vi "SaveCoords.vi"(9 "Epoch Tel":dbl=2008.731741 caption="Époque" format="%.2f", 10 "DEC Tel":dbl=70342.56719999999 caption="Ascension Droite du Télescope" format="%<%H:%M:%S%1u>t", 11 "RA Tel":dbl=70342.56719999999 caption="Ascension Droite du Télescope" format="%<%H:%M:%S%1u>t") -> (0 "Accepted?":bool, 1 "Epoch Out":dbl=2008.731741 caption="Époque" format="%.2f", 2 "DEC Out":dbl=70342.56719999999 caption="Ascension Droite du Télescope" format="%<%H:%M:%S%1u>t", 3 "RA Out":dbl=70342.56719999999 caption="Ascension Droite du Télescope" format="%<%H:%M:%S%1u>t")   [LabVIEW 2019]
panel:
  in  "Undo":bool
  in  "Save":bool
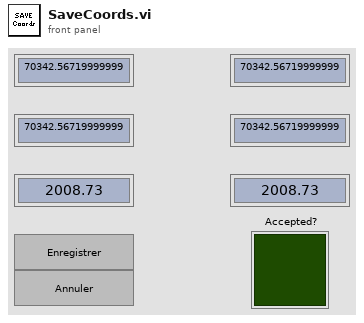
[diagram p1: front panel]
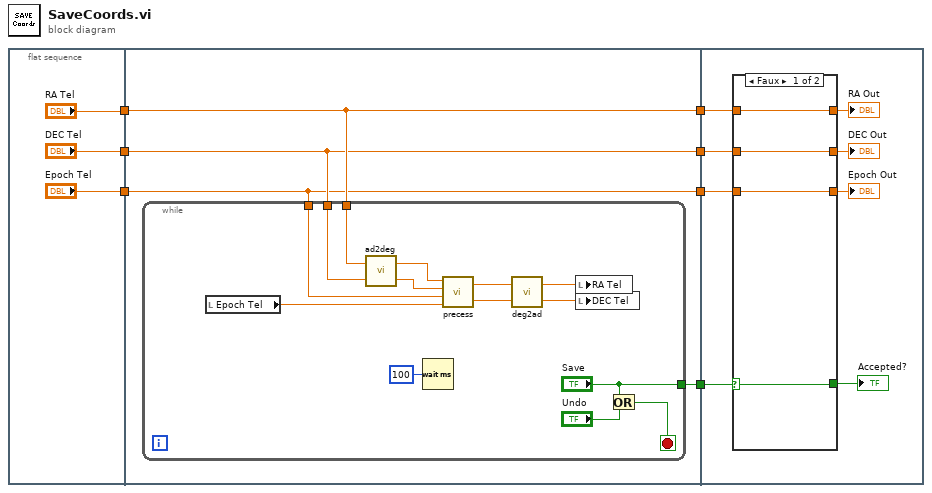
[diagram p0: block diagram]
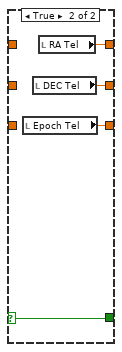
[diagram p2: hidden frame]
diagram:
  n1 = flat-sequence {
    tunnel: ["Epoch Tel"] -> w7
    tunnel: ["DEC Tel"] -> w6
    tunnel: ["RA Tel"] -> w5
    tunnel: w7 -> [w12]
    tunnel: w6 -> [w13]
    tunnel: w5 -> [w14]
    tunnel: [w12] -> w4
    tunnel: [w13] -> w3
    tunnel: [w14] -> w2
    tunnel: [w11] -> w1
    tunnel: w4 -> [w36]
    tunnel: w3 -> [w34]
    tunnel: w2 -> [w32]
    tunnel: w1 -> [w30]
    frame #0 {
    }
    frame #1 {
      n2 = while {
        tunnel: w14 -> [w20]
        tunnel: w13 -> [w19]
        tunnel: w12 -> [w26]
        tunnel: ["Save"] -> w11
        stop <- w27 stop-if-true
        n3 = local read "Epoch Tel"() -> (w25:dbl)
        n4 = call "ad2deg.vi"("DEC (sec)"=w19, "RA (sec)"=w20) -> ("DEC (°)"=w18:dbl, "RA (°)"=w17:dbl)
        n5 = Wait (ms)(milliseconds to wait=u32 100) -> ()  [unwired: 1 out]
        n6 = call "precess.vi"("Eq2"=w25, "Eq1"=w26, "DEC 1"=w18, "RA 1"=w17) -> ("DEC 2"=w21:dbl, "RA 2"=w24:dbl)
        n7 = call "deg2ad.vi"("DEC (°)"=w21, "RA (°)"=w24) -> ("DEC (°)"=w22:dbl, "RA (sec)"=w23:dbl)
        n8 = local write "RA Tel"(w23) -> ()
        n9 = local write "DEC Tel"(w22) -> ()
        n10 = Or(x="Save", y="Undo") -> (x .or. y?=w27:bool)
      }
    }
    frame #2 {
      n11 = case shown="Faux" w30 {
        selector: w30 -> [w37 w41]
        tunnel: w36 -> [w40 _]
        tunnel: [w40 w42] -> w35
        tunnel: w34 -> [w39 _]
        tunnel: [w39 w43] -> w33
        tunnel: w32 -> [w38 _]
        tunnel: [w38 w44] -> w31
        tunnel: [w37 w41] -> w29
        frame False {
        }
        frame True {
          n12 = local read "Epoch Tel"() -> (w42:dbl)
          n13 = local read "DEC Tel"() -> (w43:dbl)
          n14 = local read "RA Tel"() -> (w44:dbl)
        }
      }
      "RA Out" <- w31
      "DEC Out" <- w33
      "Epoch Out" <- w35
      "Accepted?" <- w29
    }
  }
